vi "Init.vi"(7 "Obj Dict":refnum<class "Object Dictionary.lvclass">, 8 "error in":errorcluster, 10 "OD Entry":refnum<class "Object Entry.lvclass">, 11 "PDO Mapping in":refnum<class "PDO Mapping.lvclass">) -> (0 "error out":errorcluster, 3 "PDO Mapping out":refnum<class "PDO Mapping.lvclass">)   [LabVIEW 2020, in "CANopen.lvlib" / "PDO Mapping.lvclass"]
uses:
  PDO Mapping.lvclass
  Object Entry/Object Entry.lvclass
  Object Dictionary/Object Dictionary.lvclass
  PDO Mapping.lvclass/PDO Mapping.ctl
  Sub Object/Sub Object.lvclass
  CANopen.lvlib
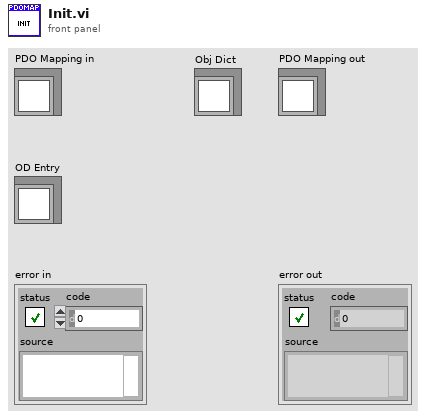
[diagram p1: front panel]
types:
  T1 = typedef "CANopen.lvlib/Access Type.ctl" = enum16{"unknown", "ro", "wo", "rw", "rwr", "rww", "const"}
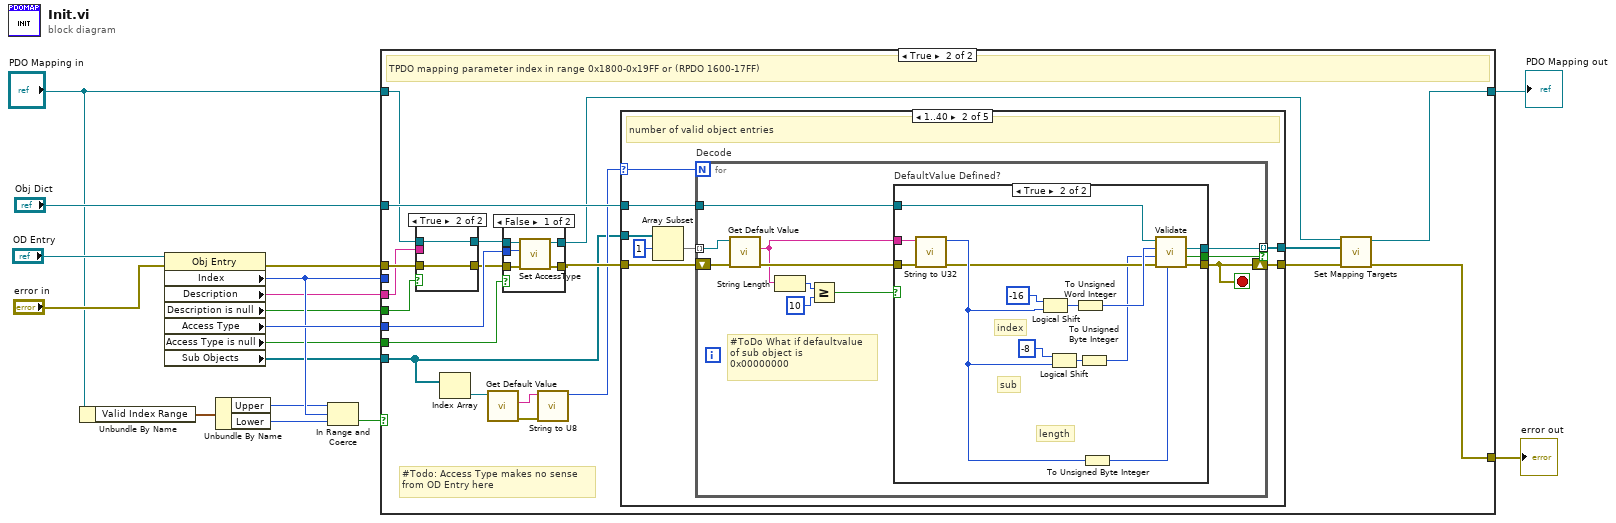
[diagram p0: block diagram]
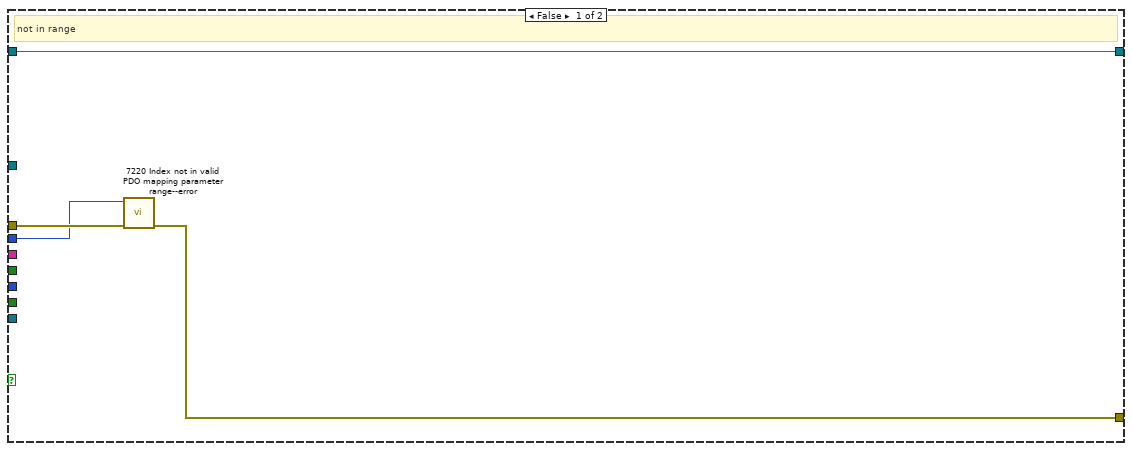
[diagram p2: hidden frame]
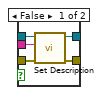
[diagram p9: hidden frame]
diagram:
  n1 = Unbundle By Name("PDO Mapping in") -> ("Valid Index Range"=w2:cluster{"Lower":u16, "Upper":u16})
  n2 = property class="Obj Entry"(reference="OD Entry", error in="error in") -> (error out=w16:errorcluster, "Index"=w14:u16, "Description"=w13:string, "Description is null"=w12:bool, "Access Type"=w17:T1, "Access Type is null"=w11:bool, "Sub Objects"=w10:refnum<class "Sub Object.lvclass">[])  [unwired: 1 out]
  n3 = Unbundle By Name(w2) -> ("Upper"=w6:u16, "Lower"=w5:u16)
  n4 = In Range and Coerce(upper limit=w6, x=w14, lower limit=w5) -> (In Range?=w15:bool)  [unwired: 1 out]
  n5 = case shown="True" w15 {
    tunnel: [w18 w41] -> w4
    tunnel: w17 -> [_ w33]
    tunnel: "PDO Mapping in" -> [w18 w37]
    tunnel: [w20 w40] -> w3
    tunnel: w16 -> [w21 w39]
    tunnel: w13 -> [_ w36]
    tunnel: "Obj Dict" -> [_ w38]
    tunnel: w10 -> [_ w22]
    tunnel: w14 -> [w19 _]
    tunnel: w12 -> [_ w35]
    tunnel: w11 -> [_ w32]
    frame False {
      # "not in range"
      n6 = call "7220 Index not in valid PDO mapping parameter range--error.vi"("error in"=w21, "Index"=w19) -> ("error out"=w20:errorcluster)  [unwired: 8 in, 1 out]
    }
    frame True {
      # "#Todo: Access Type makes no sense\nfrom OD Entry here"
      # "TPDO mapping parameter index in range 0x1800-0x19FF or (RPDO 1600-17FF)"
      n7 = case shown="True" w35 {
        tunnel: w39 -> [w93 w94]
        tunnel: [w92 w94] -> w29
        tunnel: w37 -> [w91 w95]
        tunnel: [w90 w95] -> w34
        tunnel: w36 -> [w89 _]
        frame False {
          n8 = call "Set Description.vi"("error in (no error)"=w93, "Description"=w89, "PDO Mapping in"=w91) -> ("error out"=w92:errorcluster, "PDO Mapping out"=w90:refnum<class "PDO Mapping.lvclass">)  [unwired: 7 in]
        }
        frame True {
        }
      }
      n9 = Index Array(array=w22) -> (element=w26:refnum<class "Sub Object.lvclass">)  [unwired: 1 in]
      n10 = call "Get Default Value.vi"("Sub Object in"=w26) -> ("error out"=w24:errorcluster, "Default Value"=w25:string)  [unwired: 8 in, 1 out]
      n11 = case shown="False" w32 {
        tunnel: w29 -> [w86 w87]
        tunnel: [w85 w87] -> w30
        tunnel: w34 -> [w84 w88]
        tunnel: [w83 w88] -> w31
        tunnel: w33 -> [w82 _]
        frame False {
          n12 = call "Set AccessType.vi"("error in (no error)"=w86, "AccessType"=w82, "PDO Mapping in"=w84) -> ("error out"=w85:errorcluster, "PDO Mapping out"=w83:refnum<class "PDO Mapping.lvclass">)  [unwired: 7 in]
        }
        frame True {
        }
      }
      n13 = call "String to U8.vi"("error in"=w24, "Integer String"=w25) -> ("U8"=w23:u8)  [unwired: 8 in, 1 out]
      n14 = case shown="1..40" w23 {
        selector: w23 -> [_ w46 _ _ _]
        tunnel: w38 -> [_ w50 _ _ _]
        tunnel: w30 -> [w42 w49 w79 w80 w81]
        tunnel: [w42 w48 w79 w80 w81] -> w28
        tunnel: [_ w47 _ _ _] -> w27
        tunnel: w22 -> [_ w44 _ _ _]
        frame 0, Default {
          # "Mapping disabled"
        }
        frame 1..40 {
          # "number of valid object entries"
          n15 = Array Subset(array=w44, index=1) -> (w45:refnum<class "Sub Object.lvclass">[])  [unwired: 1 in]
          n16 = for "Decode" {
            N: w46 -> [_]
            tunnel: w50 -> [w59]
            shift-right: [w56] -> w48
            shift-left: w49 -> [w61]
            tunnel: [w58] -> w47 mode=indexing if=w57
            tunnel: w45 -> [w55] mode=indexing
            stop <- w56 stop-if-true
            # "#ToDo What if defaultvalue\nof sub object is\n0x00000000"
            n17 = call "Get Default Value.vi"("error in"=w61, "Sub Object in"=w55) -> ("error out"=w60:errorcluster, "Default Value"=w54:string)  [unwired: 7 in, 1 out]
            n18 = String Length(string=w54) -> (length=w53:i32)
            n19 = Greater Or Equal?(x=w53, y=10) -> (x >= y?=w51:bool)
            n20 = case "DefaultValue Defined?" shown="True" w51 {
              selector: w51 -> [w62 _]
              tunnel: w54 -> [_ w77]
              tunnel: w60 -> [w63 w78]
              tunnel: w59 -> [_ w71]
              tunnel: [w63 w70] -> w56
              tunnel: [_ w64] -> w58
              tunnel: [w62 w65] -> w57
              frame False {
              }
              frame True {
                # "length"
                # "index"
                # "sub"
                n21 = call "String to U32.vi"("error in"=w78, "Integer String"=w77) -> ("error out"=w72:errorcluster, "U32"=w75:u32)  [unwired: 8 in]
                n22 = Logical Shift(y=i16 -16, x=w75) -> (x << y=w69:u32)
                n23 = Logical Shift(y=i16 -8, x=w75) -> (x << y=w68:u32)
                n24 = To Unsigned Word Integer(number=w69) -> (unsigned 16bit integer=w73:u16)
                n25 = To Unsigned Byte Integer(number=w68) -> (unsigned 8bit integer=w67:u8)
                n26 = To Unsigned Byte Integer(number=w75) -> (unsigned 8bit integer=w66:u8)
                n27 = call "Validate.vi"("Length"=w66, "error in"=w72, "Sub-Index"=w67, "Index"=w73, "Obj Dict"=w71) -> ("error out"=w70:errorcluster, "Valid?"=w65:bool, "Sub Obj"=w64:refnum<class "Sub Object.lvclass">)  [unwired: 4 in]
              }
            }
          }
        }
        frame 41..253 {
          # "reserved"
        }
        frame 254 {
          # "SAM-MPDO"
        }
        frame 255 {
          # "DAM-MPDO"
        }
      }
      n28 = call "Set Mapping Targets.vi"("error in (no error)"=w28, "Mapping Targets"=w27, "PDO Mapping in"=w31) -> ("error out"=w40:errorcluster, "PDO Mapping out"=w41:refnum<class "PDO Mapping.lvclass">)  [unwired: 7 in]
    }
  }
  "error out" <- w3
  "PDO Mapping out" <- w4
